vi "lua_tonumber.vi"(8 "error in (no error)":errorcluster, 10 "index":i32, 11 "lua_state_p":u64) -> (0 "error out":errorcluster, 1 "coerced?":bool, 2 "number":dbl, 3 "lua_state_p out":u64)   [LabVIEW 2020, in "lua.dll.lvlib"]
uses:
  lua.dll.lvlib
  lua54.dll
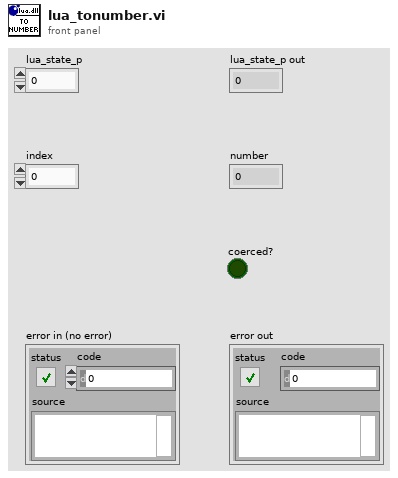
[diagram p1: front panel]
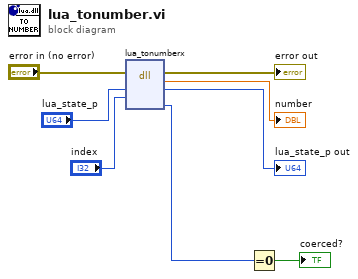
[diagram p0: block diagram]
diagram:
  n1 = dll-call lib="C:/Users/Nicholas Folse/Documents/workspace/github-tauterra.llc/Lua for LabVIEW/lib/lua.dll/lua54**.*" fn="lua_tonumberx"(error in="error in (no error)", "lua_state_p"="lua_state_p", "index"="index") -> (error out=→"error out":errorcluster, "result"=→"number":dbl, "lua_state_p"=→"lua_state_p out":u64, "isnum"=w1:i32)  [unwired: 4 in, 1 out]
  n2 = Equal To 0?(x=w1) -> (x = 0?=→"coerced?":bool)
